vi "Write.vi"(8 "error in (no error)":errorcluster, 10 "Array":string[][](array[string]), 11 "Save as ini in":refnum<class "Save as ini.lvclass">) -> (0 "error out":errorcluster, 3 "Save as ini out":refnum<class "Save as ini.lvclass">)   [LabVIEW 2020, in "Save as ini.lvclass"]
uses:
  Save as ini.lvclass
  Saving OO.lvclass
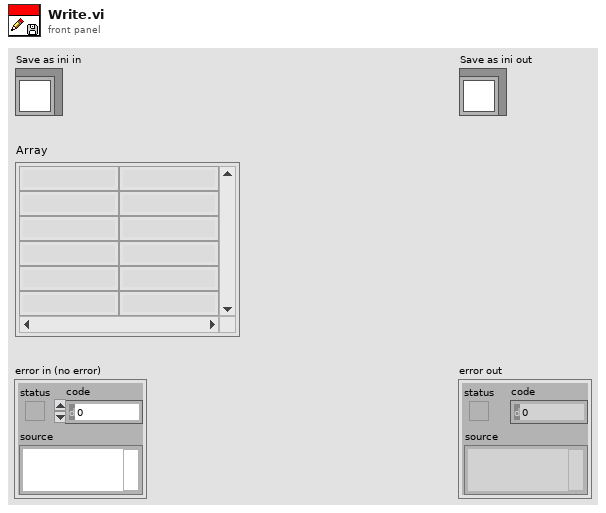
[diagram p1: front panel]
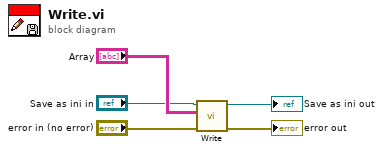
[diagram p0: block diagram]
diagram:
  n1 = call-parent "Write.vi"("error in (no error)"="error in (no error)", "Array"="Array", "Saving OO in"="Save as ini in") -> ("error out"=→"error out":errorcluster, "Saving OO out"=→"Save as ini out":refnum<class "Save as ini.lvclass">)  [unwired: 7 in]
